vi "SetupDMA.vi"(2 "blocks":u32=1, 3 "nos":u32=1, 4 "Drv":u32=1) -> ()   [LabVIEW 2017]
uses:
  ESLSCDLL.dll
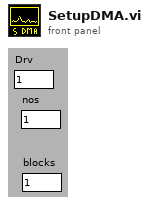
[diagram p1: front panel]
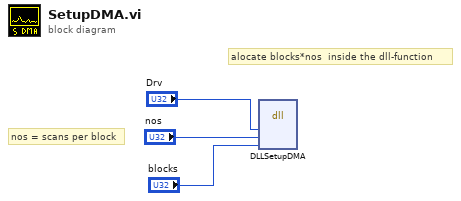
[diagram p0: block diagram]
diagram:
  # "alocate blocks*nos  inside the dll-function"
  # "nos = scans per block"
  n1 = dll-call lib="C:/ENTW/PCIE/64bit/lv64/lv64_eventdriven/board.vis/ESLSCDLL.dll" fn="DLLSetupDMA" ("lwlscdll.dll:DLLReadFFLoop")("drv"="Drv", "nos"="nos", "blocks"="blocks") -> ()  [unwired: 7 in, 2 out]
